vi "_Last Ack Queue.vi"(10 "Queue":refnum<class "Queue.lvclass">) -> (3 "Last Ack Queue Msg Strategy out":refnum<class "Last Ack Queue Msg Strategy.lvclass">)   [LabVIEW 2021, in "jettl.lvlib" / "jettl Msg Last Ack Queue.lvlib"]
uses:
  jettl Msg Last Ack Queue.lvlib
  Last Ack Queue Msg Strategy/Last Ack Queue Msg Strategy.lvclass
  Queue/Queue.lvclass
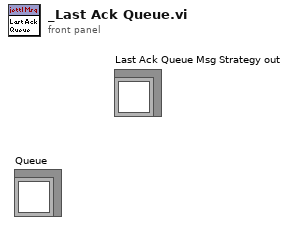
[diagram p1: front panel]
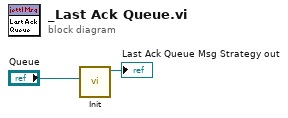
[diagram p0: block diagram]
diagram:
  n1 = call "Init.vi"("Queue"="Queue") -> ("Last Ack Queue Msg Strategy out"=→"Last Ack Queue Msg Strategy out":refnum<class "Last Ack Queue Msg Strategy.lvclass">)  [unwired: 10 in]
